vi "ColumnHeaderV2.vi"(8 "error in":errorcluster, 9 "NomDon":string[](array[string])=["RTêta;", "X&Y;"], 10 "IndCourbe":i64 caption="Numéro de Balayage", 11 "Experiment.lvclass In":refnum<class "Experiment.lvclass">) -> (0 "error out":errorcluster, 2 "Scan list":string[](array[string]), 3 "Experiment.lvclass Out":refnum<class "Experiment.lvclass">, 4 "ScanTableSize":i32[](array[numeric]))   [LabVIEW 2010, in "Experiment.lvclass"]
doc: "Ce Vi créer la ligne d'entête du fichier texte de sauvegarde à partir du nombre de courbe voulu."
uses:
  Experiment.lvclass
  Experiment.lvclass/Experiment.ctl
  DevicesClass/BaseDevice/BaseDevice.lvclass
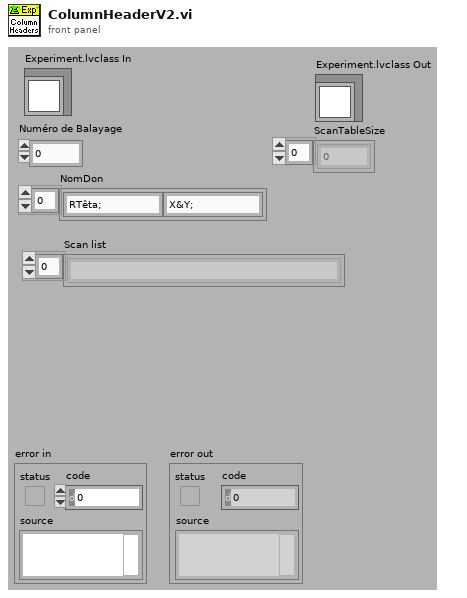
[diagram p1: front panel]
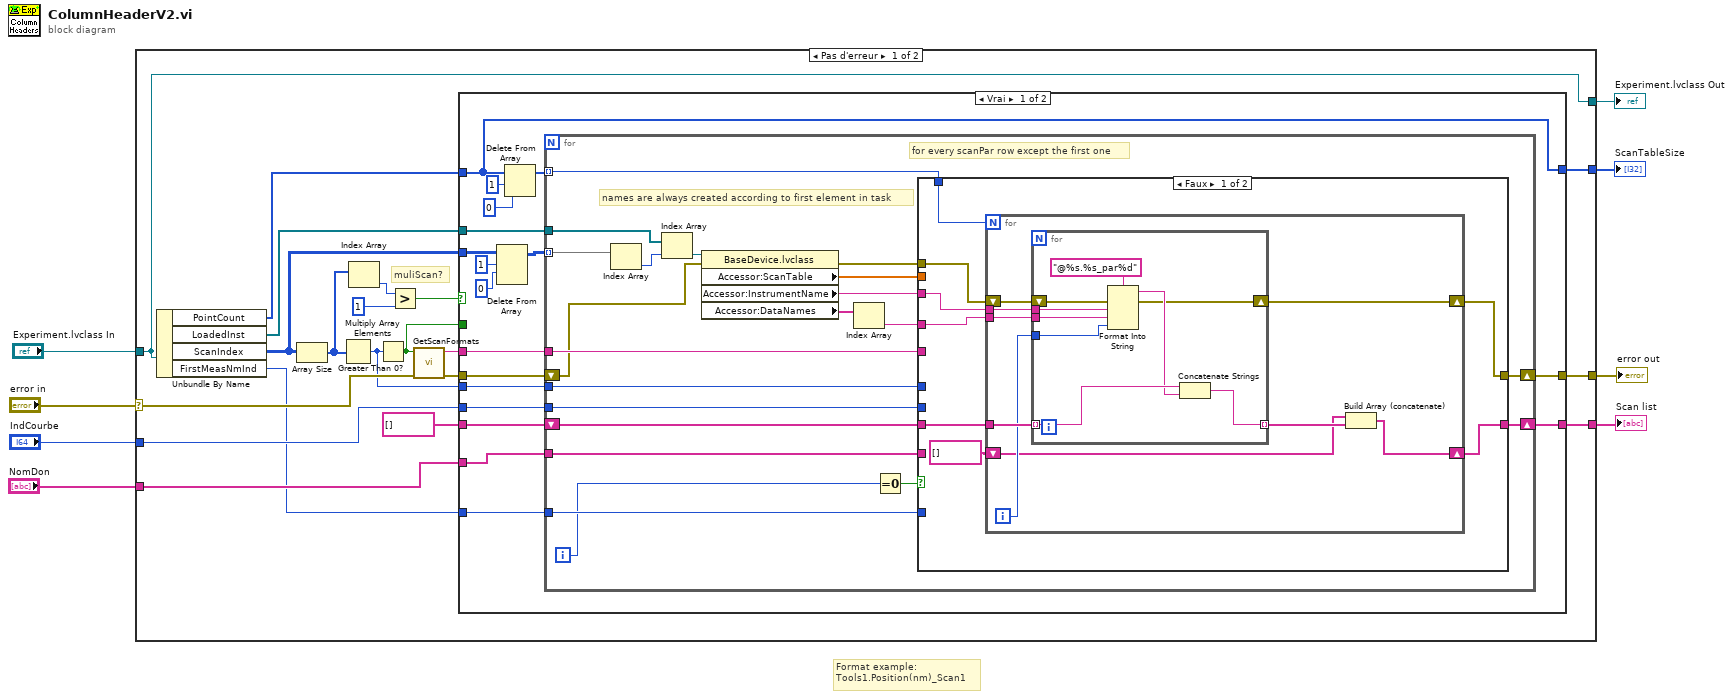
[diagram p0: block diagram]
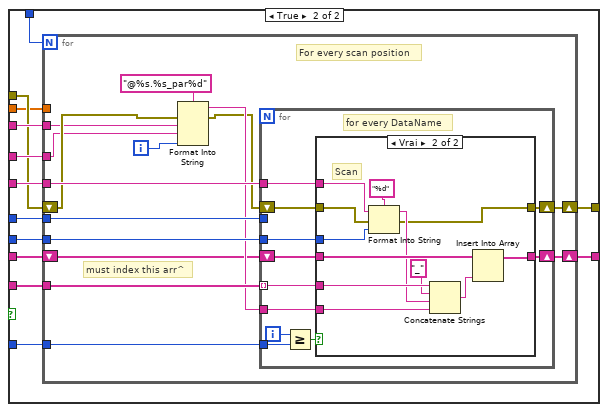
[diagram p2: hidden frame]
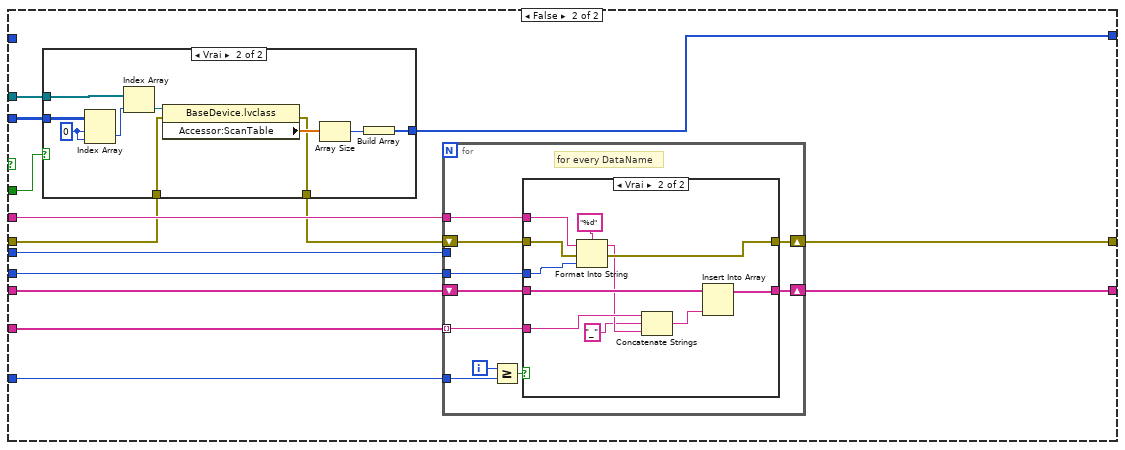
[diagram p4: hidden frame]
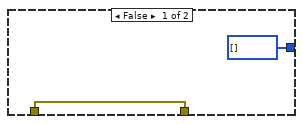
[diagram p5: hidden frame]
diagram:
  # "Format example:\nTools1.Position(nm)_Scan1"
  n1 = case shown="Pas d'erreur" "error in" {
    selector: "error in" -> [w28 w197]
    tunnel: [w17 w197] -> w7
    tunnel: [w23 _] -> w6
    tunnel: "NomDon" -> [w24 _]
    tunnel: "Experiment.lvclass In" -> [w14 w196]
    tunnel: "IndCourbe" -> [w26 _]
    tunnel: [w14 w196] -> w2
    tunnel: [w13 _] -> w1
    frame No Error {
      # "muliScan?"
      n2 = Unbundle By Name(w14) -> ("PointCount"=w9:i32[], "LoadedInst"=w18:refnum<class "BaseDevice.lvclass">[], "ScanIndex"=w19:i32[][], "FirstMeasNmInd"=w16:i32)
      n3 = Array Size(array=w19) -> (size(s)=w11:i32[])
      n4 = Multiply Array Elements(1:w11) -> (0:w21:i32)
      n5 = Index Array(array=w11) -> (element=w10:i32)  [unwired: 1 in]
      n6 = Greater Than 0?(x=w21) -> (x > 0?=w12:bool)
      n7 = Greater?(x=w10, y=1) -> (0:w15:bool)
      n8 = call "GetScanFormats.vi"("ErrorIn(No Error)"=w28, "Scan(T)"=w12) -> ("sortie d'erreur"=w25:errorcluster, "Prefixe"=w27:string)  [unwired: 7 in, 1 out]
      n9 = case shown="Vrai" w15 {
        tunnel: w27 -> [w46 w160]
        tunnel: w26 -> [w45 w159]
        tunnel: w25 -> [w44 w149]
        tunnel: w24 -> [w43 w158]
        tunnel: [w36 w157] -> w23
        tunnel: string[] [] -> [w37 w156]
        tunnel: w21 -> [w42 w155]
        tunnel: w19 -> [w41 w152]
        tunnel: w18 -> [w40 w151]
        tunnel: [w39 w154] -> w17
        tunnel: w16 -> [w38 w153]
        tunnel: [w32 w150] -> w13
        tunnel: w12 -> [_ w147]
        tunnel: w9 -> [w32 _]
        frame True {
          n10 = Delete From Array(array=w41, length=1 ("longueur"), index (row)=0 ("indice (ligne)")) -> (array with subset deleted=w35:i32[][])  [unwired: 1 in, 1 out]
          n11 = Delete From Array(array=w32, length=1 ("longueur"), index=0 ("indice")) -> (array with subset deleted=w30:i32[])  [unwired: 1 out]
          n12 = for {
            tunnel: w46 -> [w67]
            tunnel: w42 -> [w66]
            tunnel: w45 -> [w65]
            tunnel: w43 -> [w64]
            tunnel: w35 -> [w63] mode=indexing
            tunnel: w40 -> [w62]
            shift-right: [w60] -> w39
            shift-left: w44 -> [w61]
            tunnel: w38 -> [w59]
            shift-right: [w56] -> w36
            shift-left: w37 -> [w55]
            tunnel: w30 -> [w54] mode=indexing
            i -> [w47]
            # "names are always created according to first element in task"
            # "for every scanPar row except the first one"
            n13 = Index Array(array=w63) -> (element=w52:i32)  [unwired: 1 in]
            n14 = Index Array(array=w62, index=w52) -> (element=w51:refnum<class "BaseDevice.lvclass">)
            n15 = property class="BaseDevice.lvclass"(reference=w51, error in=w61) -> (error out=w53:errorcluster, "Accessor:ScanTable"=w49:dbl[], "Accessor:InstrumentName"=w57:string, "Accessor:DataNames"=w50:string[])  [unwired: 1 out]
            n16 = Index Array(array=w50) -> (element=w58:string)  [unwired: 1 in]
            n17 = Equal To 0?(x=w47) -> (x = 0?=w48:bool)
            n18 = case shown="Faux" w48 {
              tunnel: w67 -> [_ w106]
              tunnel: w66 -> [_ w105]
              tunnel: w65 -> [_ w104]
              tunnel: w64 -> [_ w103]
              tunnel: [w69 w102] -> w60
              tunnel: w59 -> [_ w101]
              tunnel: w58 -> [w74 w100]
              tunnel: w57 -> [w75 w99]
              tunnel: [w70 w98] -> w56
              tunnel: w55 -> [w72 w97]
              tunnel: w54 -> [w71 w96]
              tunnel: w53 -> [w73 w95]
              tunnel: w49 -> [_ w94]
              frame False {
                n19 = for {
                  N: w71 -> [_]
                  tunnel: w75 -> [w84]
                  tunnel: w74 -> [w83]
                  shift-right: [w78] -> w69
                  shift-left: w73 -> [w82]
                  tunnel: w72 -> [w81]
                  shift-right: [w77] -> w70
                  shift-left: string[] [] -> [w76]
                  i -> [w80]
                  n20 = for {
                    tunnel: w84 -> [w92]
                    tunnel: w83 -> [w91]
                    tunnel: w81 -> [w89] mode=indexing
                    tunnel: w80 -> [w87]
                    tunnel: [w86] -> w79 mode=indexing
                    shift-right: [w85] -> w78
                    shift-left: w82 -> [w90]
                    n21 = Format Into String(format string="@%s.%s_par%d" ("chaîne de format"), error in=w90, w92, w91, w87) -> (resulting string=w88:string, error out=w85:errorcluster)  [unwired: 1 in]
                    n22 = Concatenate Strings(w89, w88) -> (w86:string)
                  }
                  n23 = Build Array (concatenate)(w76, w79) -> (w77:string[])
                }
              }
              frame True {
                n24 = for {
                  N: w96 -> [_]
                  tunnel: w106 -> [w121]
                  tunnel: w105 -> [w120]
                  tunnel: w104 -> [w119]
                  tunnel: w103 -> [w118]
                  shift-right: [w116] -> w102
                  shift-left: w95 -> [w114]
                  tunnel: w101 -> [w115]
                  tunnel: w100 -> [w113]
                  tunnel: w99 -> [w112]
                  shift-right: [w117] -> w98
                  shift-left: w97 -> [w110]
                  tunnel: w94 -> [_]
                  i -> [w107]
                  # "must index this arr^"
                  # "For every scan position"
                  n25 = Format Into String(format string="@%s.%s_par%d" ("chaîne de format"), error in=w114, w112, w113, w107) -> (resulting string=w111:string, error out=w109:errorcluster)  [unwired: 1 in]
                  n26 = for {
                    tunnel: w121 -> [w127]
                    tunnel: w118 -> [w130] mode=indexing
                    shift-right: [w131] -> w117
                    shift-left: w110 -> [w132]
                    tunnel: w120 -> [_]
                    tunnel: w119 -> [w128]
                    shift-right: [w125] -> w116
                    shift-left: w109 -> [w126]
                    tunnel: w115 -> [w123]
                    tunnel: w111 -> [w122]
                    i -> [w124]
                    # "for every DataName"
                    n27 = Greater Or Equal?(x=w124, y=w123) -> (x >= y?=w129:bool)
                    n28 = case shown="Vrai" w129 {
                      tunnel: w132 -> [w134 w146]
                      tunnel: [w134 w145] -> w131
                      tunnel: w130 -> [_ w144]
                      tunnel: w128 -> [_ w137]
                      tunnel: w127 -> [_ w143]
                      tunnel: w126 -> [w133 w142]
                      tunnel: [w133 w135] -> w125
                      tunnel: w122 -> [_ w138]
                      frame False {
                        # "in a scan the first items are the scanpar (var param): dont include it in graph legend"
                      }
                      frame True {
                        # "Scan"
                        n29 = Format Into String(format string="%d" ("chaîne de format"), initial string=w143, error in=w142, w137) -> (resulting string=w140:string, error out=w135:errorcluster)
                        n30 = Concatenate Strings(w144, "_" ("chaîne"), w140, w138) -> (w141:string)
                        n31 = Insert Into Array(array=w146, new element=w141) -> (w145:string[])  [unwired: 1 in]
                      }
                    }
                  }
                }
              }
            }
          }
        }
        frame False {
          n32 = case shown="Vrai" w147 {
            tunnel: w152 -> [_ w170]
            tunnel: w151 -> [_ w168]
            tunnel: [i32[] [] w165] -> w150
            tunnel: w149 -> [w162 w164]
            tunnel: [w162 w163] -> w148
            frame False {
            }
            frame True {
              w169 = 0 ("indice (ligne)")
              n33 = Index Array(array=w170, index (row)=w169, index (col)=w169) -> (element=w172:i32)
              n34 = Index Array(array=w168, index=w172) -> (element=w171:refnum<class "BaseDevice.lvclass">)
              n35 = property class="BaseDevice.lvclass"(reference=w171, error in=w164) -> (error out=w163:errorcluster, "Accessor:ScanTable"=w167:dbl[])  [unwired: 1 out]
              n36 = Array Size(array=w167) -> (size(s)=w166:i32)
              n37 = Build Array(w166) -> (w165:i32[])
            }
          }
          n38 = for {
            tunnel: w160 -> [w177]
            tunnel: w158 -> [w180] mode=indexing
            shift-right: [w181] -> w157
            shift-left: w156 -> [w182]
            tunnel: w155 -> [_]
            tunnel: w159 -> [w178]
            shift-right: [w175] -> w154
            shift-left: w148 -> [w176]
            tunnel: w153 -> [w173]
            i -> [w174]
            # "for every DataName"
            n39 = Greater Or Equal?(x=w174, y=w173) -> (x >= y?=w179:bool)
            n40 = case shown="Vrai" w179 {
              tunnel: w182 -> [w184 w195]
              tunnel: [w184 w194] -> w181
              tunnel: w180 -> [_ w193]
              tunnel: w178 -> [_ w186]
              tunnel: w177 -> [_ w192]
              tunnel: w176 -> [w183 w191]
              tunnel: [w183 w190] -> w175
              frame False {
                # "in a scan the first items are the scanpar (var param): dont include it in graph legend"
              }
              frame True {
                n41 = Format Into String(format string="%d" ("chaîne de format"), initial string=w192, error in=w191, w186) -> (resulting string=w188:string, error out=w190:errorcluster)
                n42 = Concatenate Strings(w193, "_" ("chaîne"), w188) -> (w189:string)
                n43 = Insert Into Array(array=w195, new element=w189) -> (w194:string[])  [unwired: 1 in]
              }
            }
          }
        }
      }
    }
    frame Error {
    }
  }
  "error out" <- w7
  "Scan list" <- w6
  "Experiment.lvclass Out" <- w2
  "ScanTableSize" <- w1
